vi "Dispersion measurements.vi"() -> ()   [LabVIEW 2015]
uses:
  <vilib>/express/express arith-compare/Formula/XNode/ExpressFormulaBlockNode.xnode
  <instrlib>/Rohde&Schwarz Vector Network Analyzer/Rohde&Schwarz Vector Network Analyzer.lvlib
panel:
  out "Amplifier LinMag gain":dbl
  in  "Power amplifier LinMag gain (if 0, it will be calculated)":dbl min=0.0 max=20.0
  in  "Stop frequency (Hz)":dbl=15000000000.0 min=0.0 max=20000000000.0
  in  "Start frequency (Hz)":dbl=100000.0 min=0.0 max=20000000000.0
  in  "1 Hz < IFBW < 1MHz (10 kHz default)":dbl=10000.0 min=1.0 max=10000000.0
  in  "-20 dB < Power < 20 dB (0 dB default)":dbl min=-20.0 max=20.0
  in  "Delay time along ther sample (ps)":dbl min=0.0 max=1000.0
  out "DMM reading":dbl=5.649249
  out "Current field point":i32=98
  in  "DMM's connection":refnum<visa-resource-name>="Multimeter"
  in  "Choose the folder where the field dependencies of S-parameters and Z will be saved":path=path "C:/Users/ZJUcomposite/Desktop/Tests"
  in  "HMF's connection":refnum<visa-resource-name>="Generator"
  in  "VNA's connection":refnum<visa-resource-name>="ZNB-VNA"
  in  "Coil resistance > 0 (Ohm)":dbl=8.38 min=0.0 max=1000.0
  in  "Coil inductance > 0 (H)":dbl=0.32 min=0.0 max=100.0
  in  "Number of field points":i32=1 min=1 max=1000 step=1
  in  "Volltage to field coefficient > 0 (Oe/V)":dbl=4.29 min=0.0 max=1000.0
  in  "Max input voltage for the amplifier (0<V<2)":dbl=1.5 min=0.0 max=10.0
  in  "Number of frequency points":i32=5000 min=3 max=20000
  in  "VNA's port(s) used for measurements":string(combo)="S21"
  # "The procedure measures the frequency dispersions of S-parameters and Z for the specified magnetic fields.\n\nVNA must be already calibrated before the measurements. The procedure will not change the calibration but you can   modify IFBW and power. \n\nThe field values will be entered during the user dialog. All field values must be within the maximum (+/-) field range.\n\nThe voltage to field coefficient (Oe/V) must be found from the coil calibration.\n\nThe delay time along the sample must be found separately.\n\nThe coil resistance R and inductance L must be larger than zero. Measure them by a digital multimeter (DMM).\n\nPlease check the maximum input voltage max V allowed for your waveform amplifier. Also the ratio maxV / R must be below the current rate of your waveform amplifier. \n\n******************************************\nDmitriy Makhnovskiy@Hangzhou December 2018\nSensing Materials Technology Ltd, UK\nE-mail: contact@sensmattech.co.uk"
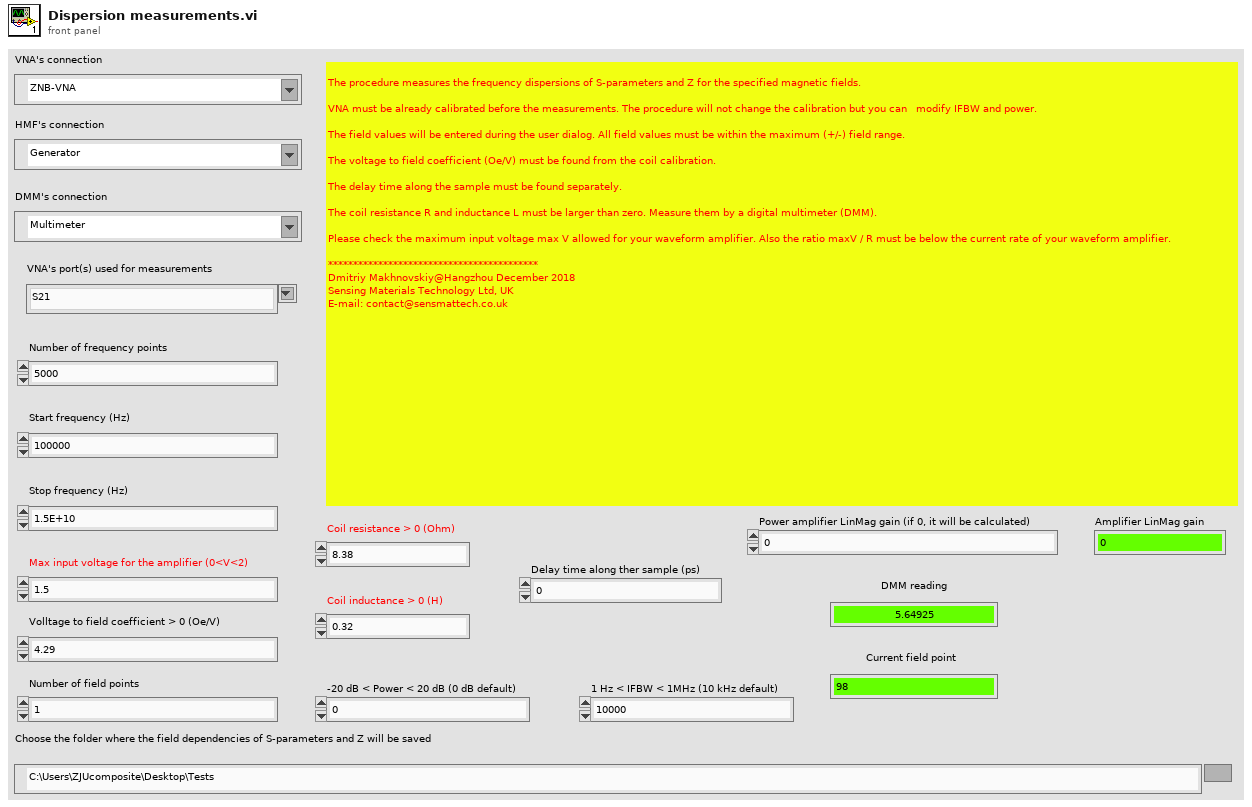
[diagram p1: front panel]
types:
  T1 = typedef "NI_Matrix.lvlib/RealMatrix.ctl" = dbl[][]
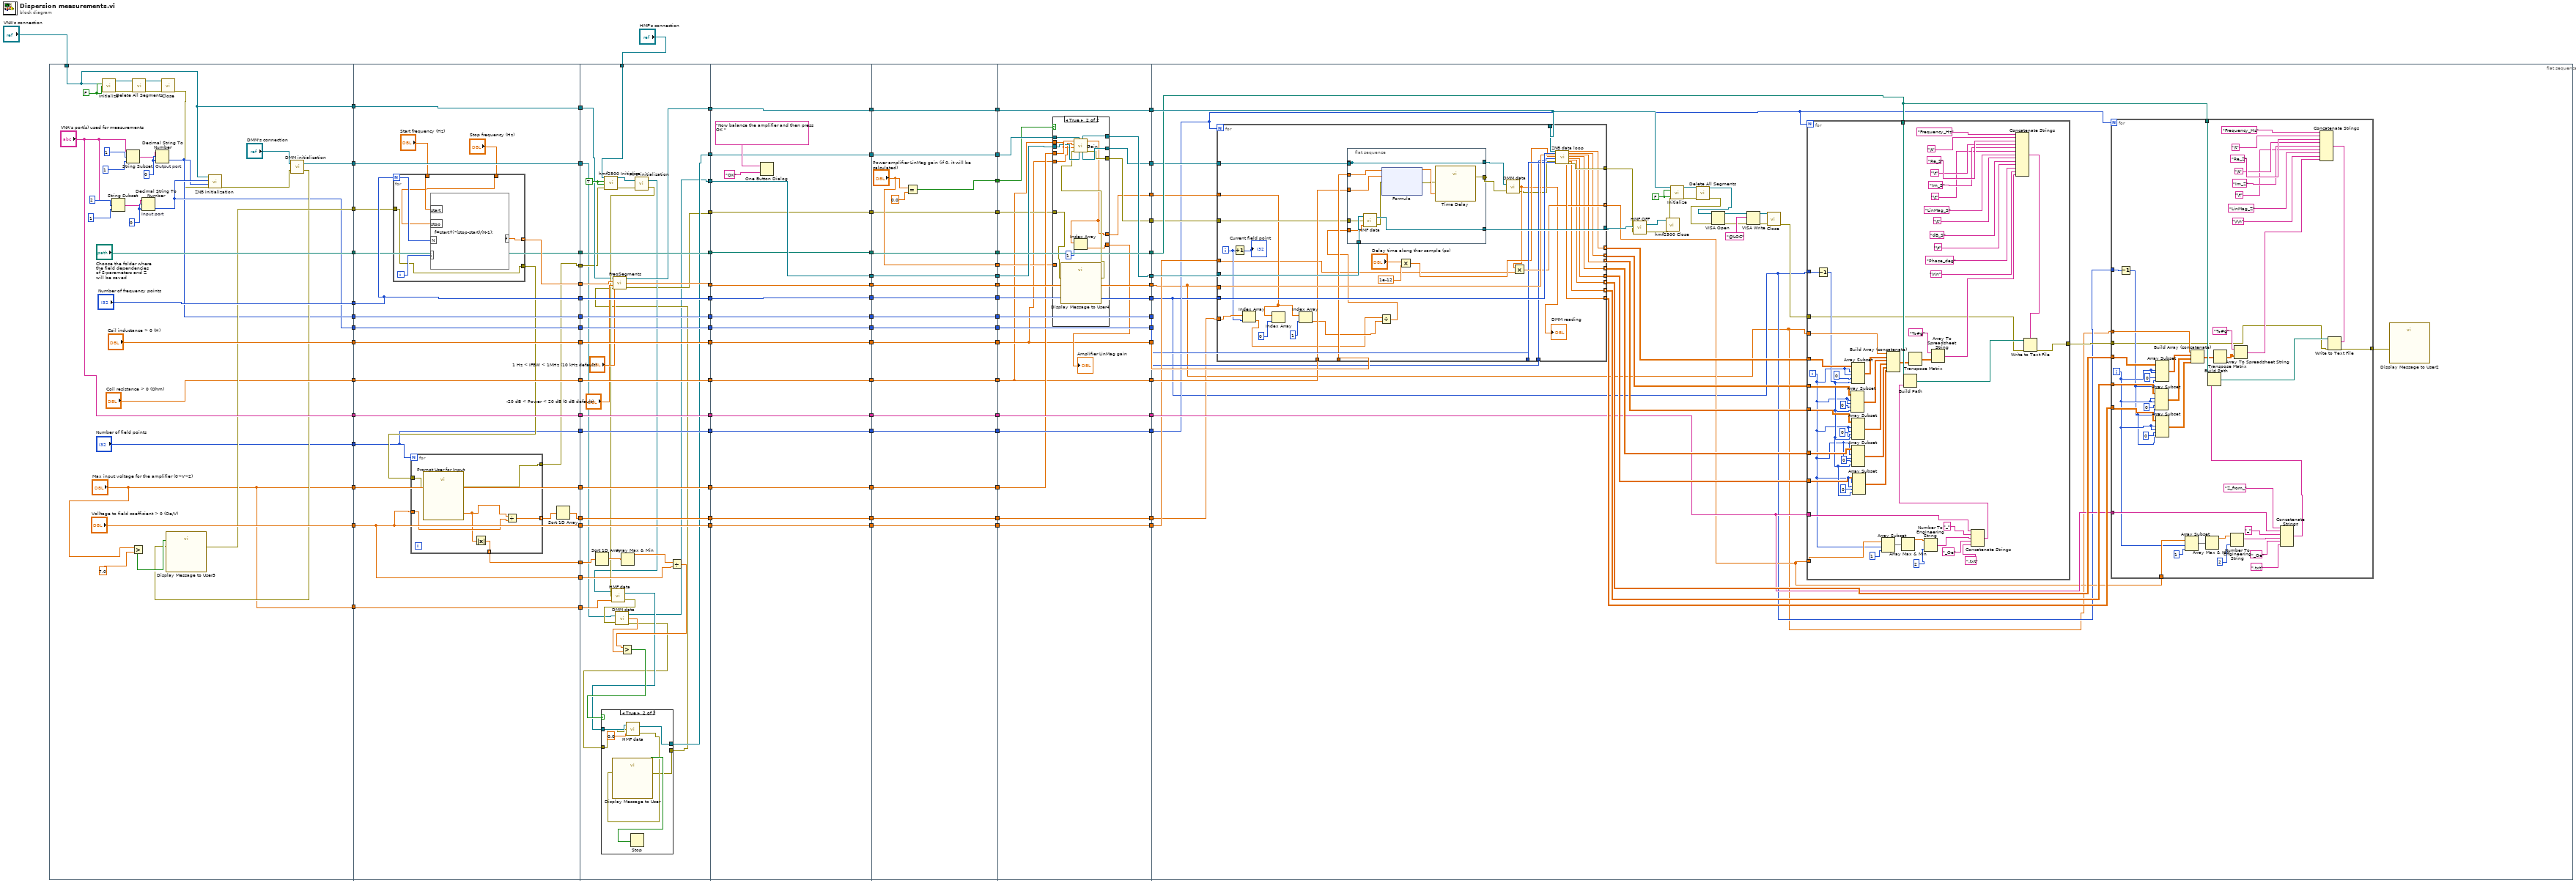
[diagram p0: block diagram]
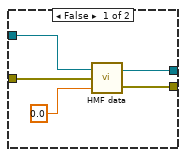
[diagram p2: hidden frame]
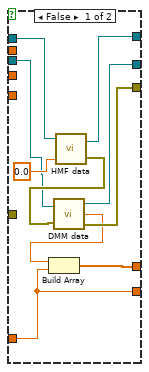
[diagram p3: hidden frame]
diagram:
  n1 = flat-sequence {
    tunnel: [w108] -> w92
    tunnel: ["VNA's port(s) used for measurements"] -> w89
    tunnel: "VNA's connection" -> [w108]
    tunnel: ["Number of frequency points"] -> w87
    tunnel: ["Coil inductance > 0 (H)"] -> w84
    tunnel: ["Coil resistance > 0 (Ohm)"] -> w81
    tunnel: ["Max input voltage for the amplifier (0<V<2)"] -> w78
    tunnel: ["Volltage to field coefficient > 0 (Oe/V)"] -> w75
    tunnel: ["Choose the folder where the field dependencies of S-parameters and Z will be saved"] -> w72
    tunnel: [w118] -> w71
    tunnel: [w113] -> w68
    tunnel: [w111] -> w65
    tunnel: [w110] -> w62
    tunnel: ["Number of field points"] -> w61
    tunnel: ["Max input voltage for the amplifier (0<V<2)"] -> w53
    tunnel: [w154] -> w100
    tunnel: [w151] -> w98
    tunnel: [w133] -> w96
    tunnel: [w153] -> w93
    tunnel: w92 -> [w153]
    tunnel: [w152] -> w90
    tunnel: w89 -> [w152]
    tunnel: w87 -> [w151]
    tunnel: [w150] -> w85
    tunnel: w84 -> [w150]
    tunnel: [w149] -> w82
    tunnel: w81 -> [w149]
    tunnel: [w137] -> w79
    tunnel: w78 -> [w137]
    tunnel: [w135] -> w76
    tunnel: w75 -> [w135]
    tunnel: [w148] -> w73
    tunnel: w72 -> [w148]
    tunnel: w71 -> [w144]
    tunnel: [w147] -> w69
    tunnel: w68 -> [w147]
    tunnel: [w146] -> w66
    tunnel: w65 -> [w146]
    tunnel: [w145] -> w63
    tunnel: w62 -> [w145]
    tunnel: w61 -> [w140]
    tunnel: [w140] -> w59
    tunnel: [w138] -> w57
    tunnel: [w136] -> w56
    tunnel: [w135] -> w55
    tunnel: [w134] -> w54
    tunnel: w53 -> [w134]
    tunnel: w100 -> [w194]
    tunnel: [w193] -> w99
    tunnel: w98 -> [w206]
    tunnel: [w206] -> w97
    tunnel: w96 -> [w174]
    tunnel: [w168] -> w95
    tunnel: [w192] -> w94
    tunnel: w93 -> [w176]
    tunnel: [w202] -> w91
    tunnel: w90 -> [w202]
    tunnel: "HMF's connection" -> [w175]
    tunnel: [w201] -> w86
    tunnel: w85 -> [w201]
    tunnel: [w200] -> w83
    tunnel: w82 -> [w200]
    tunnel: [w199] -> w80
    tunnel: w79 -> [w199]
    tunnel: [w198] -> w77
    tunnel: w76 -> [w198]
    tunnel: [w197] -> w74
    tunnel: w73 -> [w197]
    tunnel: [w178] -> w70
    tunnel: w69 -> [w170]
    tunnel: [w196] -> w67
    tunnel: w66 -> [w196]
    tunnel: [w195] -> w64
    tunnel: w63 -> [w195]
    tunnel: [w189] -> w60
    tunnel: w59 -> [w189]
    tunnel: [w188] -> w58
    tunnel: w57 -> [w188]
    tunnel: w56 -> [w185]
    tunnel: w55 -> [w184]
    tunnel: w54 -> [w182]
    tunnel: [w172] -> w3
    tunnel: w99 -> [w234]
    tunnel: [w234] -> w36
    tunnel: w97 -> [w233]
    tunnel: [w233] -> w34
    tunnel: w95 -> [w232]
    tunnel: [w232] -> w32
    tunnel: [w231] -> w30
    tunnel: w94 -> [w231]
    tunnel: [w230] -> w28
    tunnel: w91 -> [w230]
    tunnel: [w229] -> w26
    tunnel: w86 -> [w229]
    tunnel: [w228] -> w24
    tunnel: w83 -> [w228]
    tunnel: [w227] -> w22
    tunnel: w80 -> [w227]
    tunnel: [w226] -> w20
    tunnel: w77 -> [w226]
    tunnel: [w225] -> w18
    tunnel: w74 -> [w225]
    tunnel: [w224] -> w16
    tunnel: w70 -> [w224]
    tunnel: [w223] -> w14
    tunnel: w67 -> [w223]
    tunnel: [w222] -> w12
    tunnel: w64 -> [w222]
    tunnel: [w221] -> w10
    tunnel: w60 -> [w221]
    tunnel: [w220] -> w8
    tunnel: w58 -> [w220]
    tunnel: w3 -> [w219]
    tunnel: [w219] -> w2
    tunnel: w36 -> [w255]
    tunnel: [w255] -> w35
    tunnel: w34 -> [w254]
    tunnel: [w254] -> w33
    tunnel: w32 -> [w253]
    tunnel: [w253] -> w31
    tunnel: w30 -> [w252]
    tunnel: [w252] -> w29
    tunnel: w28 -> [w251]
    tunnel: [w251] -> w27
    tunnel: w26 -> [w250]
    tunnel: [w250] -> w25
    tunnel: w24 -> [w249]
    tunnel: [w249] -> w23
    tunnel: w22 -> [w248]
    tunnel: [w248] -> w21
    tunnel: w20 -> [w247]
    tunnel: [w247] -> w19
    tunnel: w18 -> [w246]
    tunnel: [w246] -> w17
    tunnel: w16 -> [w245]
    tunnel: [w245] -> w15
    tunnel: w14 -> [w244]
    tunnel: [w244] -> w13
    tunnel: w12 -> [w243]
    tunnel: [w243] -> w11
    tunnel: w10 -> [w242]
    tunnel: [w242] -> w9
    tunnel: w8 -> [w241]
    tunnel: [w241] -> w7
    tunnel: [w239] -> w6
    tunnel: ["Power amplifier LinMag gain (if 0, it will be calculated)"] -> w5
    tunnel: w2 -> [w237]
    tunnel: [w237] -> w1
    tunnel: w35 -> [w278]
    tunnel: [w278] -> w52
    tunnel: w33 -> [w277]
    tunnel: [w277] -> w51
    tunnel: w31 -> [w267]
    tunnel: [w265] -> w50
    tunnel: w29 -> [w276]
    tunnel: [w276] -> w49
    tunnel: w27 -> [w275]
    tunnel: [w275] -> w48
    tunnel: w25 -> [w257]
    tunnel: [w257] -> w47
    tunnel: w23 -> [w256]
    tunnel: [w256] -> w46
    tunnel: w21 -> [w266]
    tunnel: w19 -> [w274]
    tunnel: [w274] -> w45
    tunnel: w17 -> [w273]
    tunnel: [w273] -> w44
    tunnel: w15 -> [w268]
    tunnel: [w260] -> w43
    tunnel: w13 -> [w272]
    tunnel: [w272] -> w42
    tunnel: w11 -> [w271]
    tunnel: [w271] -> w41
    tunnel: w9 -> [w270]
    tunnel: [w270] -> w40
    tunnel: w7 -> [w269]
    tunnel: [w269] -> w39
    tunnel: [w264] -> w38
    tunnel: [w263] -> w37
    tunnel: w6 -> [w261]
    tunnel: w5 -> [w259]
    tunnel: w1 -> [w258]
    tunnel: w52 -> [w302]
    tunnel: w51 -> [w303]
    tunnel: w50 -> [w344]
    tunnel: w49 -> [w335]
    tunnel: w48 -> [w322]
    tunnel: w47 -> [w320]
    tunnel: w46 -> [w319]
    tunnel: w45 -> [w318]
    tunnel: w44 -> [w317]
    tunnel: w43 -> [w316]
    tunnel: w42 -> [w314]
    tunnel: w41 -> [w313]
    tunnel: w40 -> [w304]
    tunnel: w39 -> [w308]
    tunnel: w38 -> [w307]
    tunnel: w37 -> [w306]
    frame #0 {
      w124 = FALSE
      w132 = 0
      w128 = 0
      n2 = call <instrlib>:"Initialize.vi"("VISA resource name"=w108, "ID Query (T: Check)"=w124, "Reset (T: Reset)"=w124) -> ("VISA resource name out"=w104:refnum<visa-resource-name>, "error out"=w106:errorcluster)  [unwired: 11 in]
      n3 = String Subset(string="VNA's port(s) used for measurements", offset (0)=2, length (rest)=1) -> (substring=w131:string)
      n4 = String Subset(string="VNA's port(s) used for measurements", offset (0)=1, length (rest)=1) -> (substring=w127:string)
      n5 = Greater?(x="Max input voltage for the amplifier (0<V<2)", y=7.0) -> (0:w116:bool)
      n6 = call <instrlib>:"Delete All Segments.vi"("error in (no error)"=w106, "VISA resource name"=w104) -> ("error out"=w105:errorcluster, "VISA resource name out"=w103:refnum<visa-resource-name>)  [unwired: 8 in]
      n7 = Decimal String To Number "Input port"(string=w131, offset=w132, default (0L)=w132) -> (number=w111:i32)  [unwired: 1 out]
      n8 = Decimal String To Number "Output port"(string=w127, offset=w128, default (0L)=w128) -> (number=w110:i32)  [unwired: 1 out]
      n9 = call <instrlib>:"Close.vi"("error in (no error)"=w105, "VISA resource name"=w103) -> ("error out"=w107:errorcluster)  [unwired: 9 in]
      n10 = call "ZNB initialization.vi"("error in (no error)"=w107, "Output port"=w110, "Input port"=w111, "VISA resource name"=w108) -> ("error out"=w109:errorcluster)  [unwired: 7 in]
      n11 = call "DMM initialization.vi"("error in (no error)"=w109, "VISA resource name"="DMM's connection") -> ("error out"=w112:errorcluster, "VISA resource name out"=w113:refnum<visa-resource-name>)
      n12 = call "Display Message to User3"("error in (no error)"=w112, "Enable"=w116) -> ("error out"=w118:errorcluster)  [unwired: 8 in, 1 out]
    }
    frame #1 {
      n13 = for {
        N: w151 -> [w165]
        tunnel: [w164] -> w154 mode=indexing
        tunnel: w144 -> [w161]
        tunnel: "Start frequency (Hz)" -> [w163]
        tunnel: "Stop frequency (Hz)" -> [w162]
        tunnel: [w161] -> w141
        i -> [w166]
        n14 = formula code="f=start+i*(stop-start)/(N-1);"("start"=w163, "stop"=w162, "N"=w165, "i"=w166) -> ("f"=w164:dbl)
      }
      n15 = for {
        N: w140 -> [_]
        tunnel: w141 -> [w160]
        tunnel: w135 -> [w159]
        tunnel: [w158] -> w139 mode=indexing
        tunnel: [w156] -> w136 mode=indexing
        tunnel: [w155] -> w133
        n16 = call "Prompt User for Input"("error in (no error)"=w160) -> ("Field (Oe)"=w157:dbl, "error out"=w155:errorcluster)  [unwired: 16 in, 1 out]
        n17 = Absolute Value(x=w157) -> (abs(x)=w156:dbl)
        n18 = Divide(x=w157, y=w159) -> (x/y=w158:ext)
      }
      n19 = Sort 1D Array(array=w139) -> (sorted array=w138:ext[])
    }
    frame #2 {
      w205 = TRUE
      n20 = Sort 1D Array(array=w185) -> (sorted array=w186:dbl[])
      n21 = call <instrlib>:"hmf2500 Initialize.vi"("error in (no error)"=w174, "Reset (Reset)"=w205, "ID Query (Check)"=w205, "VISA resource name"=w175) -> ("error out"=w203:errorcluster, "VISA resource name out"=w204:refnum<visa-resource-name>)  [unwired: 6 in]
      n22 = Array Max & Min(array=w186) -> (max value=w187:dbl)  [unwired: 3 out]
      n23 = call "HMF initialization.vi"("error in (no error)"=w203, "VISA resource name"=w204) -> ("error out"=w183:errorcluster, "VISA resource name out"=w177:refnum<visa-resource-name>)
      n24 = call "HMF data.vi"("DC offset"=w182, "error in (no error)"=w183, "VISA resource name"=w177) -> ("error out"=w171:errorcluster, "VISA resource name out"=w179:refnum<visa-resource-name>)
      n25 = call "DMM data.vi"("VISA resource name"=w170, "error in (no error)"=w171) -> ("VISA resource name out"=w168:refnum<visa-resource-name>, "Voltage"=w169:dbl, "error out"=w167:errorcluster)
      n26 = Divide(x=w187, y=w184) -> (x/y=w181:dbl)
      n27 = Greater?(x=w181, y=w169) -> (0:w180:bool)
      n28 = case shown="True" w180 {
        tunnel: w179 -> [w210 w218]
        tunnel: w167 -> [w207 w215]
        tunnel: [w209 w212] -> w178
        tunnel: [w208 w213] -> w173
        frame False {
          n29 = call "HMF data.vi"("DC offset"=0.0, "error in (no error)"=w207, "VISA resource name"=w210) -> ("error out"=w208:errorcluster, "VISA resource name out"=w209:refnum<visa-resource-name>)
        }
        frame True {
          n30 = call "HMF data.vi"("DC offset"=0.0, "error in (no error)"=w215, "VISA resource name"=w218) -> ("error out"=w214:errorcluster, "VISA resource name out"=w212:refnum<visa-resource-name>)
          n31 = call "Display Message to User"("error in (no error)"=w214) -> ("error out"=w213:errorcluster, "OK"=w216:bool)  [unwired: 9 in]
          n32 = Stop(stop? (T)=w216) -> ()
        }
      }
      n33 = call "FreqSegments.vi"("VISA resource name"=w176, "FrequenciesIn"=w194, "Power"="-20 dB < Power < 20 dB (0 dB default)", "error in (no error)"=w173, "IFBW"="1 Hz < IFBW < 1MHz (10 kHz default)") -> ("VISA resource name out"=w192:refnum<visa-resource-name>, "FrequenciesOut"=w193:dbl[], "error out"=w172:errorcluster)
    }
    frame #3 {
      n34 = One Button Dialog(message="Now balance the amplifier and then press OK ", button name ("OK")="OK") -> ()  [unwired: 1 out]
    }
    frame #4 {
      n35 = Equal?(x="Power amplifier LinMag gain (if 0, it will be calculated)", y=0.0) -> (x = y?=w239:bool)
    }
    frame #5 {
      n36 = case shown="True" w261 {
        tunnel: w268 -> [w287 w298]
        tunnel: w267 -> [w284 w296]
        tunnel: w266 -> [_ w299]
        tunnel: [w286 w297] -> w265
        tunnel: [w283 w295] -> w260
        tunnel: [w282 w294] -> w264
        tunnel: [w279 w292] -> w263
        tunnel: [w280 w291] -> w262
        tunnel: w259 -> [w280 _]
        tunnel: w258 -> [_ w300]
        tunnel: w257 -> [_ w290]
        tunnel: w256 -> [_ w289]
        frame False {
          n37 = call "HMF data.vi"("DC offset"=0.0, "VISA resource name"=w287) -> ("error out"=w285:errorcluster, "VISA resource name out"=w286:refnum<visa-resource-name>)  [unwired: 1 in]
          n38 = call "DMM data.vi"("VISA resource name"=w284, "error in (no error)"=w285) -> ("VISA resource name out"=w283:refnum<visa-resource-name>, "Voltage"=w281:dbl, "error out"=w282:errorcluster)
          n39 = Build Array(w281, w280) -> (w279:dbl[])
        }
        frame True {
          n40 = call "Display Message to User4"("error in (no error)"=w300) -> ("error out"=w293:errorcluster)  [unwired: 9 in, 1 out]
          n41 = call "Gain.vi"("DMM VISA in"=w296, "HMF VISA in"=w298, "error in (no error)"=w293, "R"=w289, "L"=w290, "Max v input"=w299) -> ("error out"=w294:errorcluster, "Polynomial coeff"=w292:dbl[], "DMM VISA out"=w295:refnum<visa-resource-name>, "HMF VISA out"=w297:refnum<visa-resource-name>)  [unwired: 2 in]
          n42 = Index Array(array=w292, index=1) -> (element=w291:dbl)
        }
      }
      "Amplifier LinMag gain" <- w262
    }
    frame #6 {
      w333 = FALSE
      n43 = for {
        N: w304 -> [_]
        tunnel: w318 -> [w446]
        tunnel: w303 -> [w472]
        tunnel: [w468] -> w305 mode=indexing
        tunnel: w344 -> [w475]
        tunnel: [w474] -> w343
        tunnel: w335 -> [w473]
        tunnel: w302 -> [w471]
        tunnel: [w469] -> w323 mode=indexing
        tunnel: [w470] -> w315
        tunnel: [w467] -> w324 mode=indexing
        tunnel: [w466] -> w325 mode=indexing
        tunnel: [w465] -> w327 mode=indexing
        tunnel: [w464] -> w328 mode=indexing
        tunnel: [w463] -> w329 mode=indexing
        tunnel: [w462] -> w330 mode=indexing
        tunnel: [w461] -> w331 mode=indexing
        tunnel: w320 -> [w460]
        tunnel: w319 -> [w459]
        tunnel: w316 -> [w440]
        tunnel: w314 -> [w458]
        tunnel: w313 -> [w457]
        tunnel: w308 -> [w452]
        tunnel: w307 -> [w450]
        tunnel: w306 -> [w448]
        i -> [w451]
        n44 = Increment(x=w451) -> (x+1=→"Current field point":i32)
        n45 = Index Array(array=w452, index=w451) -> (element=w438:ext)
        n46 = Index Array(array=w448, index=0) -> ()  [unwired: 1 out]
        n47 = Index Array(array=w448, index=1) -> (element=w441:dbl)
        n48 = flat-sequence {
          tunnel: [w486] -> w474
          tunnel: w475 -> [w483]
          tunnel: [w482] -> w444
          tunnel: w460 -> [w481]
          tunnel: w459 -> [w480]
          tunnel: w450 -> [w478]
          tunnel: w445 -> [w477]
          tunnel: [w476] -> _
          tunnel: w440 -> [w476]
          tunnel: [w476] -> w439
          frame #0 {
            n49 = call "HMF data.vi"("DC offset"=w477, "error in (no error)"=w478, "VISA resource name"=w483) -> ("error out"=w479:errorcluster, "VISA resource name out"=w486:refnum<visa-resource-name>)
            n50 = xnode "Formula"("X1"=w481, "X2"=w480, "error in (no error)"=w479) -> ("Result"=w485:dbl, "error out"=w484:errorcluster)
            n51 = call "Time Delay"("error in (no error)"=w484, "Delay Time (s)"=w485) -> ("error out"=w482:errorcluster)  [unwired: 9 in]
          }
        }
        n52 = Divide(x=w438, y=w441) -> (x/y=w445:ext)
        n53 = Multiply(x="Delay time along ther sample (ps)", y=1e-12) -> (x*y=w454:dbl)
        n54 = call "DMM data.vi"("VISA resource name"=w439, "error in (no error)"=w444) -> ("Voltage"=w443:dbl, "error out"=w442:errorcluster)  [unwired: 1 out]
        "DMM reading" <- w443
        n55 = Multiply(x=w443, y=w446) -> (x*y=w468:ext)
        n56 = call "ZNB data loop.vi"("VISA resource name"=w473, "Number of frequency points"=w472, "Frequencies"=w471, "Delay Time"=w454, "Output Port"=w457, "Input Port"=w458, "error in (no error)"=w442) -> ("error out"=w470:errorcluster, "ReS"=w461:dbl[], "ImS"=w462:dbl[], "LinMagS"=w463:dbl[], "dBS"=w464:dbl[], "Phase"=w465:dbl[], "ReZ"=w466:dbl[], "ImZ"=w467:dbl[], "LinMagZ"=w469:dbl[])  [unwired: 12 in]
      }
      n57 = call "HMF OFF.vi"("error in (no error)"=w315, "VISA resource name"=w343) -> ("error out"=w341:errorcluster, "VISA resource name out"=w342:refnum<visa-resource-name>)
      n58 = call <instrlib>:"hmf2500 Close.vi"("error in (no error)"=w341, "VISA resource name"=w342) -> ("error out"=w334:errorcluster)  [unwired: 9 in]
      n59 = call <instrlib>:"Initialize.vi"("VISA resource name"=w335, "ID Query (T: Check)"=w333, "Reset (T: Reset)"=w333, "error in (no error)"=w334) -> ("VISA resource name out"=w311:refnum<visa-resource-name>, "error out"=w312:errorcluster)  [unwired: 10 in]
      n60 = call <instrlib>:"Delete All Segments.vi"("error in (no error)"=w312, "VISA resource name"=w311) -> ("error out"=w310:errorcluster, "VISA resource name out"=w309:refnum<visa-resource-name>)  [unwired: 8 in]
      n61 = VISA Open(error in (no error)=w310, VISA resource name=w309) -> (VISA resource name=w337:refnum<visa-resource-name>, error out=w336:errorcluster)  [unwired: 3 in]
      n62 = VISA Write(VISA resource name=w337, write buffer="@LOC", error in (no error)=w336) -> (VISA resource name out=w339:refnum<visa-resource-name>, error out=w338:errorcluster)  [unwired: 1 out]
      n63 = call <instrlib>:"Close.vi"("error in (no error)"=w338, "VISA resource name"=w339) -> ("error out"=w332:errorcluster)  [unwired: 9 in]
      n64 = for {
        N: w304 -> [_]
        tunnel: w332 -> [w390]
        tunnel: w305 -> [w436]
        tunnel: w331 -> [w437]
        tunnel: w302 -> [w433]
        tunnel: w303 -> [w429]
        tunnel: w322 -> [w402]
        tunnel: [w422] -> w326
        tunnel: w317 -> [w421]
        tunnel: w330 -> [w419]
        tunnel: w329 -> [w417]
        tunnel: w328 -> [w415]
        tunnel: w327 -> [w413]
        i -> [w394]
        n65 = Decrement(x=w429) -> (x-1=w395:i32)
        n66 = Array Subset(array=w419, index (row)=w394, length (row)=w394, index (col)=0, length (col)=w395) -> (w420:dbl[][])
        n67 = Array Subset(array=w437, index (row)=w394, length (row)=w394, index (col)=0, length (col)=w395) -> (w388:dbl[][])
        n68 = Array Subset(array=w417, index (row)=w394, length (row)=w394, index (col)=0, length (col)=w395) -> (w418:dbl[][])
        n69 = Array Subset(array=w415, index (row)=w394, length (row)=w394, index (col)=0, length (col)=w395) -> (w416:dbl[][])
        n70 = Array Subset(array=w413, index (row)=w394, length (row)=w394, index (col)=0, length (col)=w395) -> (w414:dbl[][])
        n71 = Array Subset(array=w436, index=w394, length=1) -> (w434:ext[])
        n72 = Build Array (concatenate)(w433, w388, w420, w418, w416, w414) -> (w389:T1)
        n73 = Array Max & Min(array=w434) -> (max value=w393:ext)  [unwired: 3 out]
        n74 = Transpose Matrix(1:w389) -> (0:w387:T1)
        n75 = Number To Engineering String(2:2, 4:w393) -> (0:w392:string)  [unwired: 2 in]
        n76 = Array To Spreadsheet String(array=w387, 3:"%#g") -> (spreadsheet string=w403:string)  [unwired: 1 in]
        n77 = Concatenate Strings(w402, "_", w392, "_Oe", ".txt") -> (w430:string)
        n78 = Build Path(base path=w421, name or relative path=w430) -> (appended path=w427:path)
        n79 = Concatenate Strings("Frequency_Hz", "\t", "Re_S", "\t", "Im_S", "\t", "LinMag_S", "\t", "dB_S", "\t", "Phase_deg", "\r\n", w403) -> (w426:string)
        n80 = Write to Text File(file (use dialog)=w427, text=w426, error in=w390) -> (error out=w422:errorcluster)  [unwired: 1 in, 2 out]
      }
      n81 = for {
        N: w304 -> [_]
        tunnel: w305 -> [w385]
        tunnel: w325 -> [w386]
        tunnel: w302 -> [w382]
        tunnel: w303 -> [w378]
        tunnel: w322 -> [w360]
        tunnel: [w371] -> w321
        tunnel: w317 -> [w370]
        tunnel: w324 -> [w368]
        tunnel: w323 -> [w366]
        tunnel: w326 -> [w347]
        i -> [w350]
        n82 = Decrement(x=w378) -> (x-1=w348:i32)
        n83 = Array Subset(array=w368, index (row)=w350, length (row)=w350, index (col)=0, length (col)=w348) -> (w369:dbl[][])
        n84 = Array Subset(array=w386, index (row)=w350, length (row)=w350, index (col)=0, length (col)=w348) -> (w381:dbl[][])
        n85 = Array Subset(array=w366, index (row)=w350, length (row)=w350, index (col)=0, length (col)=w348) -> (w367:dbl[][])
        n86 = Array Subset(array=w385, index=w350, length=1) -> (w383:ext[])
        n87 = Build Array (concatenate)(w382, w381, w369, w367) -> (w346:T1)
        n88 = Array Max & Min(array=w383) -> (max value=w355:ext)  [unwired: 3 out]
        n89 = Transpose Matrix(1:w346) -> (0:w345:T1)
        n90 = Number To Engineering String(2:2, 4:w355) -> (0:w354:string)  [unwired: 2 in]
        n91 = Array To Spreadsheet String(array=w345, 3:"%#g") -> (spreadsheet string=w357:string)  [unwired: 1 in]
        n92 = Concatenate Strings("Z_from_", w360, "_", w354, "_Oe", ".txt") -> (w379:string)
        n93 = Build Path(base path=w370, name or relative path=w379) -> (appended path=w376:path)
        n94 = Concatenate Strings("Frequency_Hz", "\t", "Re_Z", "\t", "Im_Z", "\t", "LinMag_Z", "\r\n", w357) -> (w375:string)
        n95 = Write to Text File(file (use dialog)=w376, text=w375, error in=w347) -> (error out=w371:errorcluster)  [unwired: 1 in, 2 out]
      }
      n96 = call "Display Message to User2"("error in (no error)"=w321) -> ()  [unwired: 9 in, 2 out]
    }
  }
